vi "Front Controller.vi"() -> ()   [LabVIEW 2017]
panel:
  out "Move Log":bool
  in  "Self-destruct Password":string
  out "Log String":string
  out "Log Activated":bool
  in  "log path (use dialog)":path
  out "Password Correct":bool
  out "Local Cooling Request":bool
  in  "Close Valve 2":timestamp format="%<%H:%M:%S>T"
  in  "Open Valve 2":timestamp format="%<%H:%M:%S>T"
  in  "Close Valve 1":timestamp format="%<%H:%M:%S>T"
  in  "Open Valve 1":timestamp format="%<%H:%M:%S>T"
  out "Movement":bool
  out "System Status":string
  in  "logout":bool
  out "Close Valve 2 LED":bool
  out "Open Valve 2 LED":bool
  out "Close Valve 1 LED":bool
  out "Open Valve 1 LED":bool
  out "System Time":timestamp format="%<%H:%M:%S>T"
  in  "address":string="localhost"
  in  "stop":bool
  in  "Username":string
  in  "Password":string
  in  "?":bool
  out "Accelerometer":cluster{dbl, dbl, dbl}(graph)
  out "Temperature":dbl(knob) scale=0.0..30.0
  # "Nuclear Cooling Interface"
  # "Temperature"
  # "Acceleration"
  # "Cooling Events"
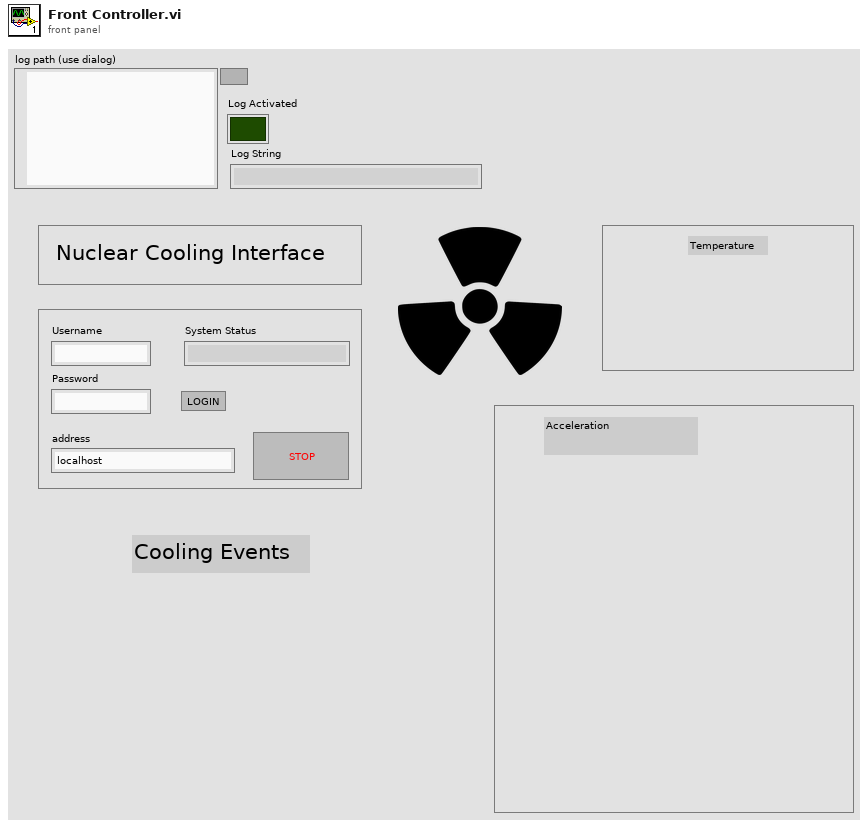
[diagram p1: front panel]
types:
  T1 = enum16{"open", "replace", "create", "open or create", "replace or create", "replace or create with confirmation"}
  T2 = cluster{"Numeric":dbl, dbl, dbl, dbl, bool, dbl, bool, dbl}
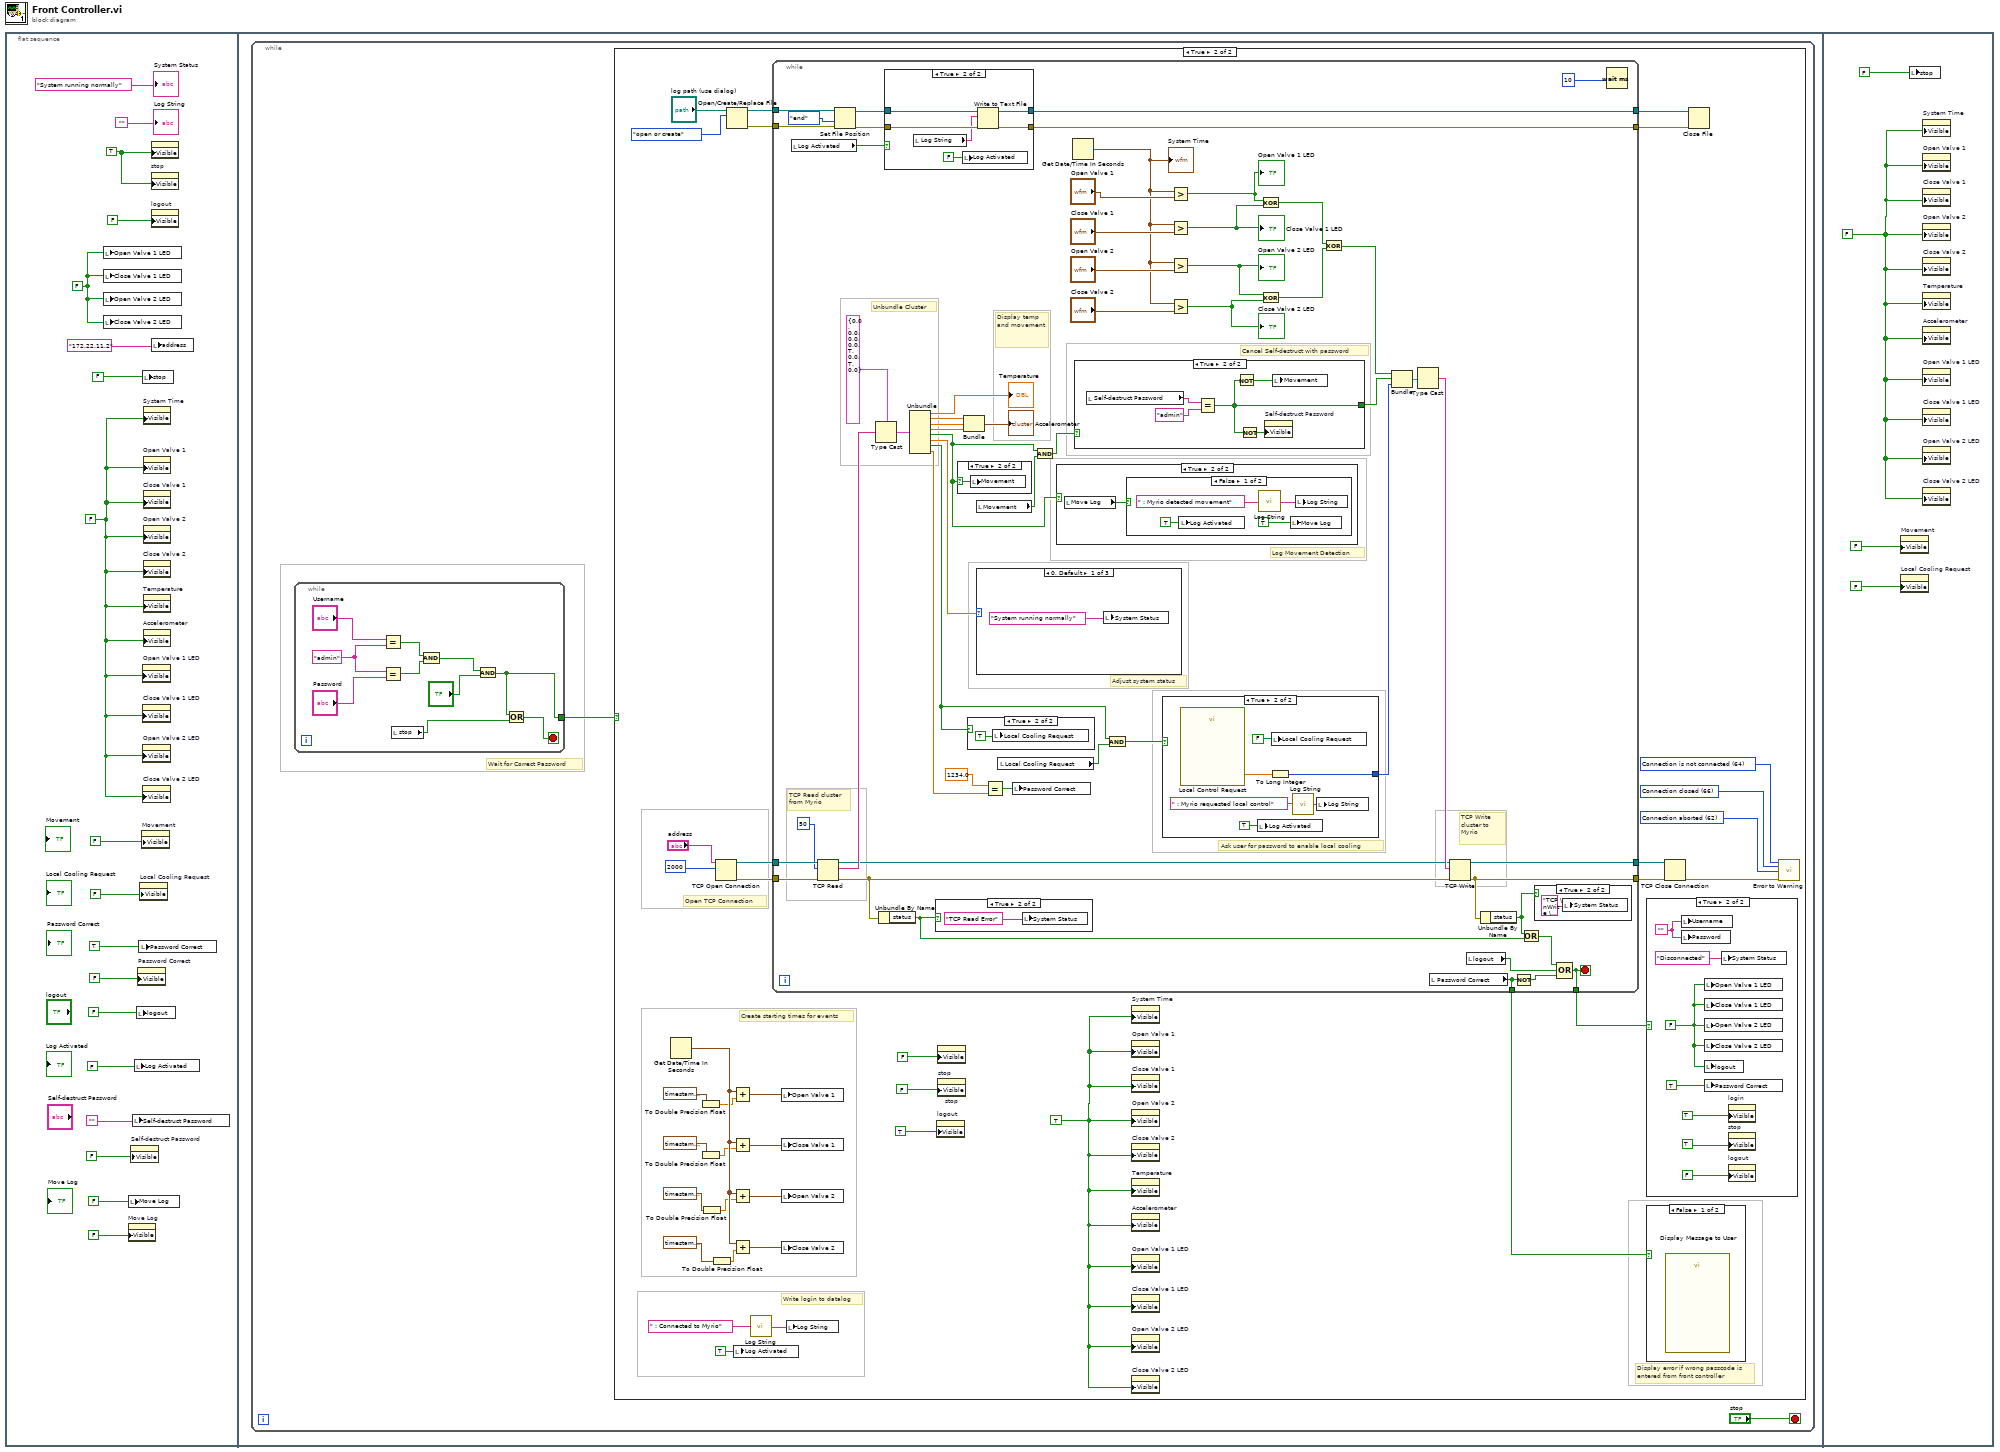
[diagram p0: block diagram]
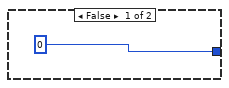
[diagram p11: hidden frame]
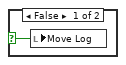
[diagram p12: hidden frame]
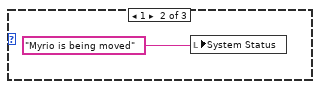
[diagram p13: hidden frame]
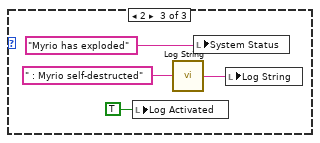
[diagram p14: hidden frame]
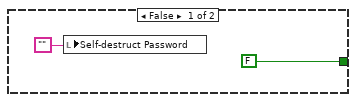
[diagram p15: hidden frame]
diagram:
  n1 = flat-sequence {
    frame #0 {
      w14 = TRUE
      w15 = FALSE
      w18 = FALSE
      n2 = local write "Open Valve 1 LED"(w18) -> ()
      n3 = local write "Close Valve 1 LED"(w18) -> ()
      n4 = local write "Open Valve 2 LED"(w18) -> ()
      n5 = local write "Close Valve 2 LED"(w18) -> ()
      n6 = local write "Move Log"(FALSE) -> ()
      n7 = property on="Move Log" class="Bool (strict)"("Visible"=FALSE) -> ()  [unwired: 2 in, 2 out]
      n8 = property on="Self-destruct Password" class="Str"("Visible"=FALSE) -> ()  [unwired: 2 in, 2 out]
      n9 = local write "Self-destruct Password"("") -> ()
      n10 = local write "Log Activated"(FALSE) -> ()
      n11 = local write "logout"(FALSE) -> ()
      n12 = property on="Password Correct" class="Bool (strict)"("Visible"=FALSE) -> ()  [unwired: 2 in, 2 out]
      n13 = local write "Password Correct"(TRUE) -> ()
      n14 = property on="Local Cooling Request" class="Bool (strict)"("Visible"=FALSE) -> ()  [unwired: 2 in, 2 out]
      n15 = property on="Movement" class="Bool (strict)"("Visible"=FALSE) -> ()  [unwired: 2 in, 2 out]
      n16 = local write "stop"(FALSE) -> ()
      n17 = property on="Open Valve 1 LED" class="Bool (strict)"("Visible"=w15) -> ()  [unwired: 2 in, 2 out]
      n18 = property on="Close Valve 1 LED" class="Bool (strict)"("Visible"=w15) -> ()  [unwired: 2 in, 2 out]
      n19 = property on="Open Valve 2 LED" class="Bool (strict)"("Visible"=w15) -> ()  [unwired: 2 in, 2 out]
      n20 = property on="Close Valve 2 LED" class="Bool (strict)"("Visible"=w15) -> ()  [unwired: 2 in, 2 out]
      n21 = property on="System Time" class="AbsTime (strict)"("Visible"=w15) -> ()  [unwired: 2 in, 2 out]
      n22 = property on="Open Valve 1" class="AbsTime (strict)"("Visible"=w15) -> ()  [unwired: 2 in, 2 out]
      n23 = property on="Close Valve 1" class="AbsTime (strict)"("Visible"=w15) -> ()  [unwired: 2 in, 2 out]
      n24 = property on="Open Valve 2" class="AbsTime (strict)"("Visible"=w15) -> ()  [unwired: 2 in, 2 out]
      n25 = property on="Close Valve 2" class="AbsTime (strict)"("Visible"=w15) -> ()  [unwired: 2 in, 2 out]
      n26 = property on="Temperature" class="Knob (strict)"("Visible"=w15) -> ()  [unwired: 2 in, 2 out]
      n27 = property on="Accelerometer" class="WFChart (strict)"("Visible"=w15) -> ()  [unwired: 2 in, 2 out]
      n28 = property class="Bool"("Visible"=w14) -> ()  [unwired: 2 in, 2 out]
      n29 = property on="stop" class="Bool (strict)"("Visible"=w14) -> ()  [unwired: 2 in, 2 out]
      n30 = property on="logout" class="Bool (strict)"("Visible"=FALSE) -> ()  [unwired: 2 in, 2 out]
      n31 = local write "address"("172.22.11.2") -> ()
      "System Status" <- "System running normally"
      "Log String" <- ""
    }
    frame #1 {
      n32 = while {
        stop <- "stop" stop-if-true
        # "Wait for Correct Password"
        n33 = while {
          tunnel: [w21] -> w19
          stop <- w22 stop-if-true
          w28 = "admin"
          n34 = Equal?(x="Username", y=w28) -> (x = y?=w27:bool)
          n35 = Equal?(x=w28, y="Password") -> (x = y?=w26:bool)
          n36 = local read "stop"() -> (w24:bool)
          n37 = And(x=w27, y=w26) -> (x .and. y?=w25:bool)
          n38 = And(x=w25, y="?") -> (x .and. y?=w21:bool)
          n39 = Or(x=w21, y=w24) -> (x .or. y?=w22:bool)
        }
        n40 = case shown="True" w19 {
          frame False {
          }
          frame True {
            w43 = TRUE
            w61 = 62 items=["No Error", "Argument Error", "Memory Full", "Out of Zone", "End of File", "File Already Open", "Generic File IO Error", "File Not Found", "File Permission Error", "Disk Full", "Duplicate Path", "Too Many Files Open", "Not Enabled", "Resource File Not Found", "Cannot Add Resource", "Resource Not Found", "Image Not Found", "Image Memory Error", "Pen Does Not Exist", "Config Bad Type", "Config Token Not Found", "Config Parse Error", "Config Memory Error", "Bad External Code Format", "Bad External Code Offset", "External Code Not Present", "Null Window", "Destroy Window Mixup", "Null Menu", "Print Aborted", "Bad Print Record", "Print Driver Error", "Windows Error During Print", "Memory Error During Print", "Print Dialog Error", "Generic Print Error", "Invalid Device Refnum", "Device Not Found", "Device Parameter Error", "Device Unit Error", "Can't Open Device", "Device Call Aborted", "Generic Error", "Cancelled By User", "Object ID Too Low", "Object ID Too High", "Object Not In Heap", "Unknown Heap", "Bad DefProc ID", "DefProc Not In Table", "Message Out Of Range", "Null Method", "Unknown Message", "Manager Call Not Supported", "Bad address", "Connection In progress", "Connection timed out", "Connection is already in progress", "Network attribute not supported", "Network error", "Address in use", "System out of memory", "Connection aborted", "Connection refused", "Connection is not connected", "Connection is already connected", "Connection closed", "Initialize error (interapplication manager)", "Bad occurrence", "Wait on unbound occurrence handler", "Occurrence queue overflow", "Bad path", "Semaphore not signaled", "Unrecognized type (interapplication manager)"] ("3rd Error to Convert")
            w62 = 66 items=["No Error", "Argument Error", "Memory Full", "Out of Zone", "End of File", "File Already Open", "Generic File IO Error", "File Not Found", "File Permission Error", "Disk Full", "Duplicate Path", "Too Many Files Open", "Not Enabled", "Resource File Not Found", "Cannot Add Resource", "Resource Not Found", "Image Not Found", "Image Memory Error", "Pen Does Not Exist", "Config Bad Type", "Config Token Not Found", "Config Parse Error", "Config Memory Error", "Bad External Code Format", "Bad External Code Offset", "External Code Not Present", "Null Window", "Destroy Window Mixup", "Null Menu", "Print Aborted", "Bad Print Record", "Print Driver Error", "Windows Error During Print", "Memory Error During Print", "Print Dialog Error", "Generic Print Error", "Invalid Device Refnum", "Device Not Found", "Device Parameter Error", "Device Unit Error", "Can't Open Device", "Device Call Aborted", "Generic Error", "Cancelled By User", "Object ID Too Low", "Object ID Too High", "Object Not In Heap", "Unknown Heap", "Bad DefProc ID", "DefProc Not In Table", "Message Out Of Range", "Null Method", "Unknown Message", "Manager Call Not Supported", "Bad address", "Connection In progress", "Connection timed out", "Connection is already in progress", "Network attribute not supported", "Network error", "Address in use", "System out of memory", "Connection aborted", "Connection refused", "Connection is not connected", "Connection is already connected", "Connection closed", "Initialize error (interapplication manager)", "Bad occurrence", "Wait on unbound occurrence handler", "Occurrence queue overflow", "Bad path", "Semaphore not signaled", "Unrecognized type (interapplication manager)"] ("2nd Error to Convert")
            w63 = 64 items=["No Error", "Argument Error", "Memory Full", "Out of Zone", "End of File", "File Already Open", "Generic File IO Error", "File Not Found", "File Permission Error", "Disk Full", "Duplicate Path", "Too Many Files Open", "Not Enabled", "Resource File Not Found", "Cannot Add Resource", "Resource Not Found", "Image Not Found", "Image Memory Error", "Pen Does Not Exist", "Config Bad Type", "Config Token Not Found", "Config Parse Error", "Config Memory Error", "Bad External Code Format", "Bad External Code Offset", "External Code Not Present", "Null Window", "Destroy Window Mixup", "Null Menu", "Print Aborted", "Bad Print Record", "Print Driver Error", "Windows Error During Print", "Memory Error During Print", "Print Dialog Error", "Generic Print Error", "Invalid Device Refnum", "Device Not Found", "Device Parameter Error", "Device Unit Error", "Can't Open Device", "Device Call Aborted", "Generic Error", "Cancelled By User", "Object ID Too Low", "Object ID Too High", "Object Not In Heap", "Unknown Heap", "Bad DefProc ID", "DefProc Not In Table", "Message Out Of Range", "Null Method", "Unknown Message", "Manager Call Not Supported", "Bad address", "Connection In progress", "Connection timed out", "Connection is already in progress", "Network attribute not supported", "Network error", "Address in use", "System out of memory", "Connection aborted", "Connection refused", "Connection is not connected", "Connection is already connected", "Connection closed", "Initialize error (interapplication manager)", "Bad occurrence", "Wait on unbound occurrence handler", "Occurrence queue overflow", "Bad path", "Semaphore not signaled", "Unrecognized type (interapplication manager)"] ("1st Error to Convert")
            # "Display error if wrong passcode is entered from front controller"
            # "Write login to datalog"
            # "Create starting times for events"
            # "Open TCP Connection"
            n41 = Get Date/Time In Seconds() -> (seconds since 1Jan1904=w55:timestamp)
            n42 = To Double Precision Float(number=timestamp(20 s since 1904-01-01)) -> (double precision float=w54:dbl)
            n43 = To Double Precision Float(number=timestamp(40 s since 1904-01-01)) -> (double precision float=w53:dbl)
            n44 = To Double Precision Float(number=timestamp(60 s since 1904-01-01)) -> (double precision float=w52:dbl)
            n45 = To Double Precision Float(number=timestamp(80 s since 1904-01-01)) -> (double precision float=w51:dbl)
            n46 = TCP Open Connection(address="address", remote port or service name=u16 2000) -> (connection ID=w67:refnum<k5>, error out=w68:errorcluster)  [unwired: 1 in, 2 out]
            n47 = Open/Create/Replace File(file path (use dialog)="log path (use dialog)", operation (0:open)=T1."open or create") -> (refnum out=w37:refnum<file>, error out=w36:errorcluster)  [unwired: 4 in, 1 out]
            n48 = Add(x=w55, y=w54) -> (x+y=w56:timestamp)
            n49 = Add(x=w55, y=w53) -> (x+y=w57:timestamp)
            n50 = Add(x=w55, y=w52) -> (x+y=w58:timestamp)
            n51 = Add(x=w55, y=w51) -> (x+y=w59:timestamp)
            n52 = local write "Log Activated"(TRUE) -> ()
            n53 = call "Log String.vi"("Message"=" : Connected to Myrio") -> ("Log String"=w33:string)
            n54 = while {
              tunnel: w68 -> [w133]
              tunnel: w67 -> [w132]
              tunnel: [w107] -> w66
              tunnel: [w120] -> w65
              tunnel: [w92] -> w41
              tunnel: [w89] -> w40
              tunnel: w37 -> [w88]
              tunnel: w36 -> [w87]
              tunnel: [w82] -> w35
              tunnel: [w81] -> w34
              stop <- w92 stop-if-true
              # "TCP Write cluster to Myrio"
              # "Ask user for password to enable local cooling"
              # "Adjust system status"
              # "Cancel Self-destruct with password"
              # "Log Movement Detection"
              # "Display temp and movement"
              # "Unbundle Cluster"
              # "TCP Read cluster\nfrom Myrio"
              n55 = local read "Log Activated"() -> (w85:bool)
              n56 = TCP Read(connection ID=w132, bytes to read=50, error in (no error)=w133) -> (connection ID out=w106:refnum<k5>, data out=w122:string, error out=w121:errorcluster)  [unwired: 1 in, 1 out]
              n57 = Set File Position(refnum=w88, from (0:start)=enum16{"start", "end", "current"}."end", error in=w87) -> (refnum out=w84:refnum<file>, error out=w83:errorcluster)  [unwired: 1 in]
              n58 = Type Cast(type=T2 {"Numeric"=0.0, 0.0, 0.0, 0.0, TRUE, 0.0, TRUE, 0.0}, x=w122) -> (*(type *) &x=w129:T2)
              n59 = Unbundle By Name(w121) -> ("status"=w78:bool)
              n60 = case shown="True" w85 {
                tunnel: w84 -> [w142 w148]
                tunnel: w83 -> [w141 w147]
                tunnel: [w142 w145] -> w82
                tunnel: [w141 w144] -> w81
                frame False {
                }
                frame True {
                  n61 = local read "Log String"() -> (w146:string)
                  n62 = local write "Log Activated"(FALSE) -> ()
                  n63 = Write to Text File(file (use dialog)=w148, text=w146, error in=w147) -> (refnum out=w145:refnum<file>, error out=w144:errorcluster)  [unwired: 1 in, 1 out]
                }
              }
              n64 = Unbundle(w129) -> ("Numeric"=→"Temperature":dbl, w127:dbl, w126:dbl, w123:dbl, w77:bool, w101:dbl, w96:bool, w94:dbl)
              n65 = case shown="True" w78 {
                frame False {
                }
                frame True {
                  n66 = local write "System Status"("TCP Read Error") -> ()
                }
              }
              n67 = case shown="True" w77 {
                selector: w77 -> [w157 w158]
                frame False {
                  n68 = local write "Move Log"(w157) -> ()
                }
                frame True {
                  n69 = local write "Movement"(w158) -> ()
                }
              }
              n70 = Bundle(w127, w126, w123) -> (→"Accelerometer":cluster{dbl, dbl, dbl})  [unwired: 1 in]
              n71 = case shown="True" w96 {
                frame False {
                }
                frame True {
                  n72 = local write "Local Cooling Request"(TRUE) -> ()
                }
              }
              n73 = local read "Movement"() -> (w102:bool)
              n74 = case shown="0, Default" w101 {
                frame 0, Default {
                  n75 = local write "System Status"("System running normally") -> ()
                }
                frame 1 {
                  n76 = local write "System Status"("Myrio is being moved") -> ()
                }
                frame 2 {
                  n77 = local write "Log Activated"(TRUE) -> ()
                  n78 = call "Log String.vi"("Message"=" : Myrio self-destructed") -> ("Log String"=w162:string)
                  n79 = local write "System Status"("Myrio has exploded") -> ()
                  n80 = local write "Log String"(w162) -> ()
                }
              }
              n81 = Equal?(x=1234.0, y=w94) -> (x = y?=w80:bool)
              n82 = local read "Local Cooling Request"() -> (w97:bool)
              n83 = local write "Password Correct"(w80) -> ()
              n84 = And(x=w77, y=w102) -> (x .and. y?=w103:bool)
              n85 = case shown="True" w77 {
                frame False {
                }
                frame True {
                  n86 = local read "Move Log"() -> (w134:bool)
                  n87 = case shown="False" w134 {
                    frame False {
                      n88 = local write "Log Activated"(TRUE) -> ()
                      n89 = call "Log String.vi"("Message"=" : Myrio detected movement") -> ("Log String"=w135:string)
                      n90 = local write "Move Log"(TRUE) -> ()
                      n91 = local write "Log String"(w135) -> ()
                    }
                    frame True {
                    }
                  }
                }
              }
              n92 = Get Date/Time In Seconds() -> (seconds since 1Jan1904=w108:timestamp)
              "System Time" <- w108
              n93 = case shown="True" w103 {
                tunnel: [FALSE w168] -> w104
                frame False {
                  n94 = local write "Self-destruct Password"("") -> ()
                }
                frame True {
                  n95 = local read "Self-destruct Password"() -> (w170:string)
                  n96 = Equal?(x=w170, y="admin") -> (x = y?=w168:bool)
                  n97 = Not(x=w168) -> (.not. x?=w167:bool)
                  n98 = Not(x=w168) -> (.not. x?=w169:bool)
                  n99 = property on="Self-destruct Password" class="Str"("Visible"=w169) -> ()  [unwired: 2 in, 2 out]
                  n100 = local write "Movement"(w167) -> ()
                }
              }
              n101 = And(x=w96, y=w97) -> (x .and. y?=w98:bool)
              n102 = case shown="True" w98 {
                tunnel: [0 w154] -> w99
                frame False {
                }
                frame True {
                  n103 = call "Local Control Request"() -> ("Passcode"=w155:dbl)  [unwired: 17 in, 2 out]
                  n104 = local write "Log Activated"(TRUE) -> ()
                  n105 = To Long Integer(number=w155) -> (32bit integer=w154:i32)
                  n106 = local write "Local Cooling Request"(FALSE) -> ()
                  n107 = call "Log String.vi"("Message"=" : Myrio requested local control") -> ("Log String"=w151:string)
                  n108 = local write "Log String"(w151) -> ()
                }
              }
              n109 = Greater?(x=w108, y="Open Valve 1") -> (0:w118:bool)
              "Open Valve 1 LED" <- w118
              n110 = Greater?(x=w108, y="Close Valve 1") -> (0:w117:bool)
              "Close Valve 1 LED" <- w117
              n111 = Greater?(x=w108, y="Open Valve 2") -> (0:w116:bool)
              "Open Valve 2 LED" <- w116
              n112 = Greater?(x=w108, y="Close Valve 2") -> (0:w115:bool)
              "Close Valve 2 LED" <- w115
              n113 = Exclusive Or(1:w117, 2:w118) -> (0:w114:bool)
              n114 = Exclusive Or(1:w115, 2:w116) -> (0:w113:bool)
              n115 = Exclusive Or(1:w113, 2:w114) -> (0:w105:bool)
              n116 = Bundle(w105, w104, w99) -> (w100:cluster{bool, bool, i32})  [unwired: 1 in]
              n117 = Type Cast(x=w100) -> (*(type *) &x=w119:string)  [unwired: 1 in]
              n118 = local read "Password Correct"() -> (w89:bool)
              n119 = TCP Write(connection ID=w106, data in=w119, error in (no error)=w121) -> (connection ID out=w120:refnum<k5>, error out=w107:errorcluster)  [unwired: 1 in, 1 out]
              n120 = local read "logout"() -> (w90:bool)
              n121 = Unbundle By Name(w107) -> ("status"=w79:bool)
              n122 = Not(x=w89) -> (.not. x?=w91:bool)
              n123 = Or(x=w79, y=w78) -> (x .or. y?=w93:bool)
              n124 = case shown="True" w79 {
                frame False {
                }
                frame True {
                  n125 = local write "System Status"("TCP \nWrite \nError") -> ()
                }
              }
              n126 = Compound Arithmetic op=OR(w93, w90, w91) -> (w92:bool)
              n127 = Wait (ms)(milliseconds to wait=u32 10) -> ()  [unwired: 1 out]
            }
            n128 = local write "Open Valve 1"(w56) -> ()
            n129 = local write "Close Valve 1"(w57) -> ()
            n130 = local write "Open Valve 2"(w58) -> ()
            n131 = local write "Close Valve 2"(w59) -> ()
            n132 = local write "Log String"(w33) -> ()
            n133 = property on="logout" class="Bool (strict)"("Visible"=TRUE) -> ()  [unwired: 2 in, 2 out]
            n134 = property class="Bool"("Visible"=FALSE) -> ()  [unwired: 2 in, 2 out]
            n135 = property on="stop" class="Bool (strict)"("Visible"=FALSE) -> ()  [unwired: 2 in, 2 out]
            n136 = property on="stop" class="Bool (strict)"("Visible"=FALSE) -> ()  [unwired: 2 in, 2 out]
            n137 = property on="System Time" class="AbsTime (strict)"("Visible"=w43) -> ()  [unwired: 2 in, 2 out]
            n138 = property on="Open Valve 1" class="AbsTime (strict)"("Visible"=w43) -> ()  [unwired: 2 in, 2 out]
            n139 = property on="Close Valve 1" class="AbsTime (strict)"("Visible"=w43) -> ()  [unwired: 2 in, 2 out]
            n140 = property on="Open Valve 2" class="AbsTime (strict)"("Visible"=w43) -> ()  [unwired: 2 in, 2 out]
            n141 = property on="Close Valve 2" class="AbsTime (strict)"("Visible"=w43) -> ()  [unwired: 2 in, 2 out]
            n142 = property on="Temperature" class="Knob (strict)"("Visible"=w43) -> ()  [unwired: 2 in, 2 out]
            n143 = property on="Accelerometer" class="WFChart (strict)"("Visible"=w43) -> ()  [unwired: 2 in, 2 out]
            n144 = property on="Open Valve 1 LED" class="Bool (strict)"("Visible"=w43) -> ()  [unwired: 2 in, 2 out]
            n145 = property on="Close Valve 1 LED" class="Bool (strict)"("Visible"=w43) -> ()  [unwired: 2 in, 2 out]
            n146 = property on="Open Valve 2 LED" class="Bool (strict)"("Visible"=w43) -> ()  [unwired: 2 in, 2 out]
            n147 = property on="Close Valve 2 LED" class="Bool (strict)"("Visible"=w43) -> ()  [unwired: 2 in, 2 out]
            n148 = case shown="True" w41 {
              frame False {
              }
              frame True {
                w71 = FALSE
                w76 = ""
                n149 = local write "Username"(w76) -> ()
                n150 = local write "Password"(w76) -> ()
                n151 = local write "Open Valve 1 LED"(w71) -> ()
                n152 = local write "Close Valve 1 LED"(w71) -> ()
                n153 = local write "Open Valve 2 LED"(w71) -> ()
                n154 = local write "Close Valve 2 LED"(w71) -> ()
                n155 = local write "logout"(w71) -> ()
                n156 = local write "Password Correct"(TRUE) -> ()
                n157 = local write "System Status"("Disconnected") -> ()
                n158 = property on="login" class="Bool"("Visible"=TRUE) -> ()  [unwired: 2 in, 2 out]
                n159 = property on="stop" class="Bool (strict)"("Visible"=TRUE) -> ()  [unwired: 2 in, 2 out]
                n160 = property on="logout" class="Bool (strict)"("Visible"=FALSE) -> ()  [unwired: 2 in, 2 out]
              }
            }
            n161 = case shown="False" w40 {
              frame False {
                n162 = call "Display Message to User"() -> ()  [unwired: 10 in, 2 out]
              }
              frame True {
              }
            }
            n163 = TCP Close Connection(connection ID=w65, error in (no error)=w66) -> (error out=w64:errorcluster)  [unwired: 2 out]
            n164 = Close File(refnum=w35, error in=w34) -> ()  [unwired: 2 out]
            n165 = call <vilib>:"Error to Warning.vi"("1st Error to Convert"=w63, "2nd Error to Convert"=w62, "3rd Error to Convert"=w61, "error in"=w64) -> ()  [unwired: 2 in, 10 out]
          }
        }
      }
    }
    frame #2 {
      w174 = FALSE
      n166 = property on="Movement" class="Bool (strict)"("Visible"=FALSE) -> ()  [unwired: 2 in, 2 out]
      n167 = property on="Local Cooling Request" class="Bool (strict)"("Visible"=FALSE) -> ()  [unwired: 2 in, 2 out]
      n168 = local write "stop"(FALSE) -> ()
      n169 = property on="System Time" class="AbsTime (strict)"("Visible"=w174) -> ()  [unwired: 2 in, 2 out]
      n170 = property on="Open Valve 1" class="AbsTime (strict)"("Visible"=w174) -> ()  [unwired: 2 in, 2 out]
      n171 = property on="Close Valve 1" class="AbsTime (strict)"("Visible"=w174) -> ()  [unwired: 2 in, 2 out]
      n172 = property on="Open Valve 2" class="AbsTime (strict)"("Visible"=w174) -> ()  [unwired: 2 in, 2 out]
      n173 = property on="Close Valve 2" class="AbsTime (strict)"("Visible"=w174) -> ()  [unwired: 2 in, 2 out]
      n174 = property on="Temperature" class="Knob (strict)"("Visible"=w174) -> ()  [unwired: 2 in, 2 out]
      n175 = property on="Accelerometer" class="WFChart (strict)"("Visible"=w174) -> ()  [unwired: 2 in, 2 out]
      n176 = property on="Open Valve 1 LED" class="Bool (strict)"("Visible"=w174) -> ()  [unwired: 2 in, 2 out]
      n177 = property on="Close Valve 1 LED" class="Bool (strict)"("Visible"=w174) -> ()  [unwired: 2 in, 2 out]
      n178 = property on="Open Valve 2 LED" class="Bool (strict)"("Visible"=w174) -> ()  [unwired: 2 in, 2 out]
      n179 = property on="Close Valve 2 LED" class="Bool (strict)"("Visible"=w174) -> ()  [unwired: 2 in, 2 out]
    }
  }
